vi "Check Number of Elements in all Worker Queues.vi"(11 "CheckAll_WKR_Queues in":refnum<class "_Check all Worker Queues.lvclass">) -> (3 "Array":string[][](array[string]))   [LabVIEW 2017, in "_Check all Worker Queues.lvclass"]
uses:
  _Check all Worker Queues.lvclass
  C:/Program Files (x86)/National Instruments/LabVIEW 2017/vi.lib/addons/_Workers/Library/Classes/Worker/Worker.lvclass
  <vilib>/addons/_Workers/Library/Classes/Worker/Worker.lvclass/Worker.ctl
  <vilib>/addons/_Workers/Library/Classes/Worker/Worker.lvclass
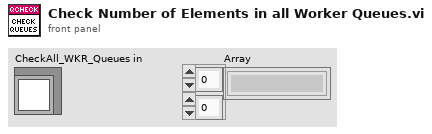
[diagram p1: front panel]
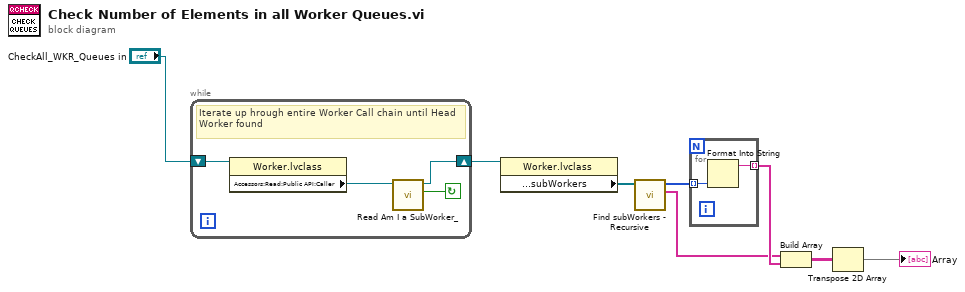
[diagram p0: block diagram]
diagram:
  n1 = while {
    shift-right: [w9] -> w1
    shift-left: "CheckAll_WKR_Queues in" -> [w12]
    stop <- w11 continue-if-true
    # "Iterate up hrough entire Worker Call chain until Head Worker found"
    n2 = property class="Worker.lvclass"(reference=w12) -> ("Accessors:Read:Public API:Caller"=w10:refnum<class "Worker.lvclass">)  [unwired: 1 in, 2 out]
    n3 = call <vilib>:"Read Am I a SubWorker_.vi"("Worker"=w10) -> ("Am I a SubWorker?"=w11:bool, "Worker out"=w9:refnum<class "Worker.lvclass">)  [unwired: 9 in]
  }
  n4 = property class="Worker.lvclass"(reference=w1) -> ("Accessors:Read:Public API:subWorkers"=w2:refnum<class "Worker.lvclass">[])  [unwired: 1 in, 2 out]
  n5 = call "Find subWorkers - Recursive.vi"("subWorkers"=w2) -> ("WIDs"=w4:string[], "Elements in Queue"=w3:i32[])  [unwired: 9 in]
  n6 = for {
    tunnel: w3 -> [w14] mode=indexing
    tunnel: [w13] -> w5 mode=indexing
    n7 = Format Into String(w14) -> (resulting string=w13:string)  [unwired: 3 in, 1 out]
  }
  n8 = Build Array(w4, w5) -> (w6:string[][])
  n9 = Transpose 2D Array(2D array=w6) -> (transposed array=→"Array":string[][])
